vi "NI-RFSG_Open.vi"(8 "error in":errorcluster, 10 "Reset?":bool=TRUE, 11 "Alias":string) -> (0 "error out":errorcluster {"code" format="%.0x"}, 3 "Handle":variant)   [LabVIEW 2015]
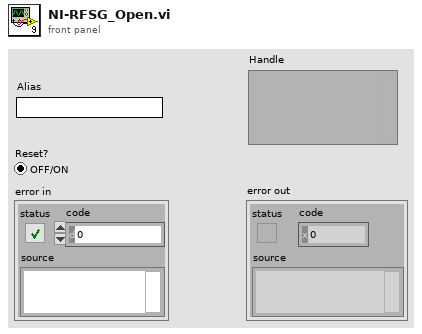
[diagram p1: front panel]
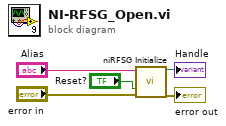
[diagram p0: block diagram]
diagram:
  n1 = call <instrlib>:"niRFSG Initialize.vi"("resource name"="Alias", "reset device"="Reset?", "error in"="error in") -> ("instrument handle"=→"Handle":refnum<k15>, "error out"=→"error out":errorcluster)  [unwired: 11 in]
